vi "QUADBIFUR.vi"() -> ()   [LabVIEW 2012]
panel:
  in  "Number of Iterates \nper value of R":dbl=100.0
  out "Bifurcation Diagram of Quadratic Map":cluster{dbl[], "Array of Xn":dbl[]}(graph)
  out "Progress":dbl(slide) scale=0.0..1.0
  in  "# of values between start\nand stop":i32=200
  in  "R Stop":dbl=3.7
  in  "R Start":dbl=3.0
  in  "Number of Pre-Iterates":dbl=100.0
  # "THE QUADRATIC MAP: XN+1 = RXN(1-XN)"
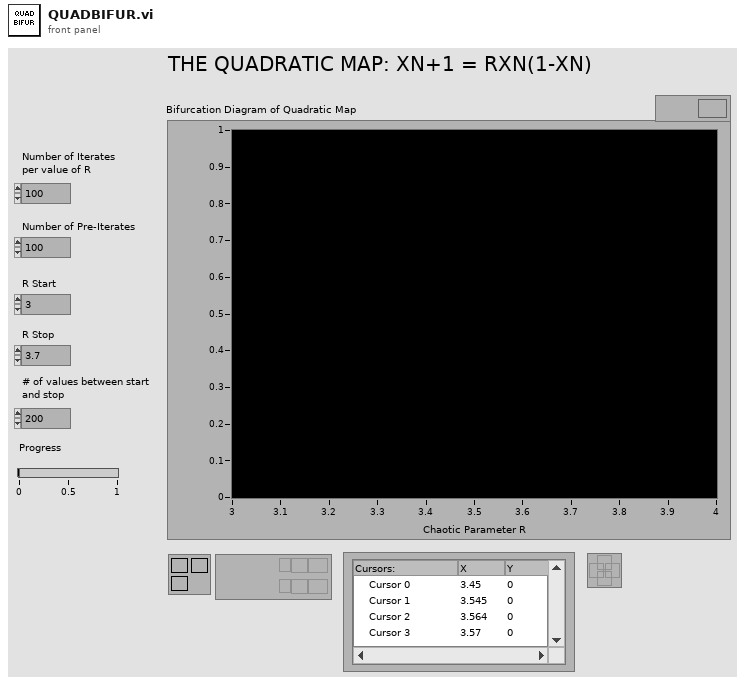
[diagram p1: front panel]
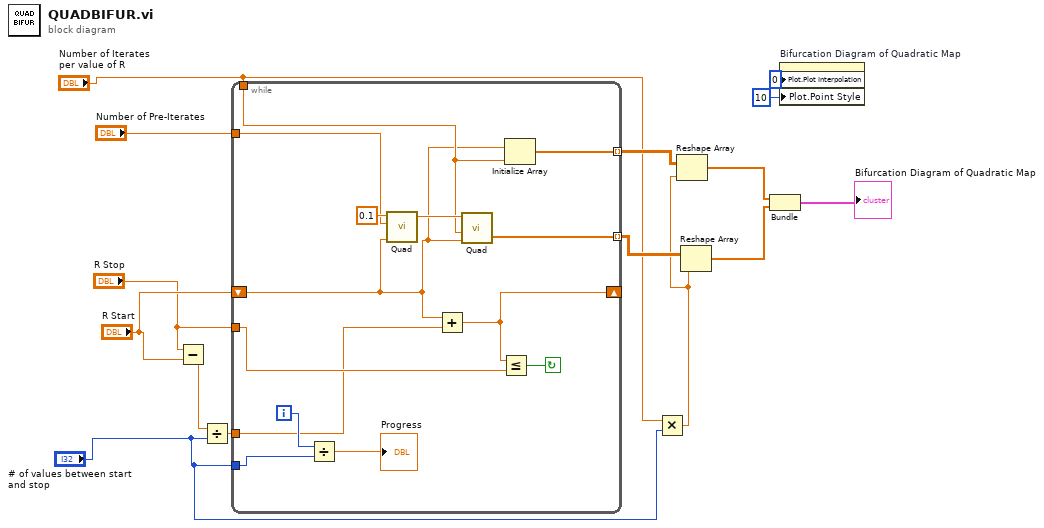
[diagram p0: block diagram]
diagram:
  n1 = Subtract(x="R Stop", y="R Start") -> (x-y=w13:dbl)
  n2 = Divide(x=w13, y="# of values between start\nand stop") -> (x/y=w12:dbl)
  n3 = while {
    tunnel: "Number of Iterates \nper value of R" -> [w23]
    tunnel: "Number of Pre-Iterates" -> [w28]
    shift-right: [w16] -> _
    shift-left: "R Start" -> [w19]
    tunnel: w12 -> [w18]
    tunnel: "# of values between start\nand stop" -> [w25]
    tunnel: [w22] -> w8 mode=indexing
    tunnel: [w21] -> w9 mode=indexing
    tunnel: "R Stop" -> [w20]
    i -> [w26]
    stop <- w17 continue-if-true
    n4 = Divide(x=w26, y=w25) -> (x/y=→"Progress":dbl)
    n5 = call "Quad.vi"("Chaotic parameter"=w19, "Number of pre-iterates"=w28, "Initial Value"=0.1) -> ("Final iterate"=w27:dbl)  [unwired: 1 in, 1 out]
    n6 = Add(x=w19, y=w18) -> (x+y=w16:dbl)
    n7 = call "Quad.vi"("Chaotic parameter"=w19, "Number of Iterates to compute"=w23, "Initial Value"=w27) -> ("Array of Xn"=w21:dbl[])  [unwired: 1 in, 1 out]
    n8 = Less Or Equal?(x=w16, y=w20) -> (x <= y?=w17:bool)
    n9 = Initialize Array(w19, w23) -> (w22:dbl[])
  }
  n10 = Multiply(x="Number of Iterates \nper value of R", y="# of values between start\nand stop") -> (x*y=w7:dbl)
  n11 = Reshape Array(w8, w7) -> (w6:dbl[])
  n12 = Reshape Array(w9, w7) -> (w5:dbl[])
  n13 = Bundle(w6, "Array of Xn"=w5) -> (→"Bifurcation Diagram of Quadratic Map":cluster{dbl[], "Array of Xn":dbl[]})  [unwired: 1 in]
  n14 = property on="Bifurcation Diagram of Quadratic Map" class="XYGraph (strict)"("Plot.Plot Interpolation"=u8 0, "Plot.Point Style"=u8 10) -> ()  [unwired: 2 in, 2 out]
